vi "GetGPIBName.vi"(8 "Error In":errorcluster, 9 "GPIB ID":u32=1 min=1 step=1, 10 "GPIB Board":u32 min=1 step=1, 11 "VISA Resource List":string[](array[string])) -> (0 "Error Out":errorcluster, 2 "Found?":bool, 3 "VISA GPIB Resource Name":string)   [LabVIEW 2013, in "LV-Utilities.lvlib"]
uses:
  LV-Utilities.lvlib
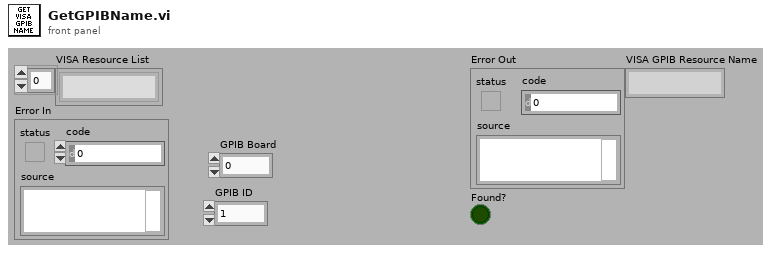
[diagram p1: front panel]
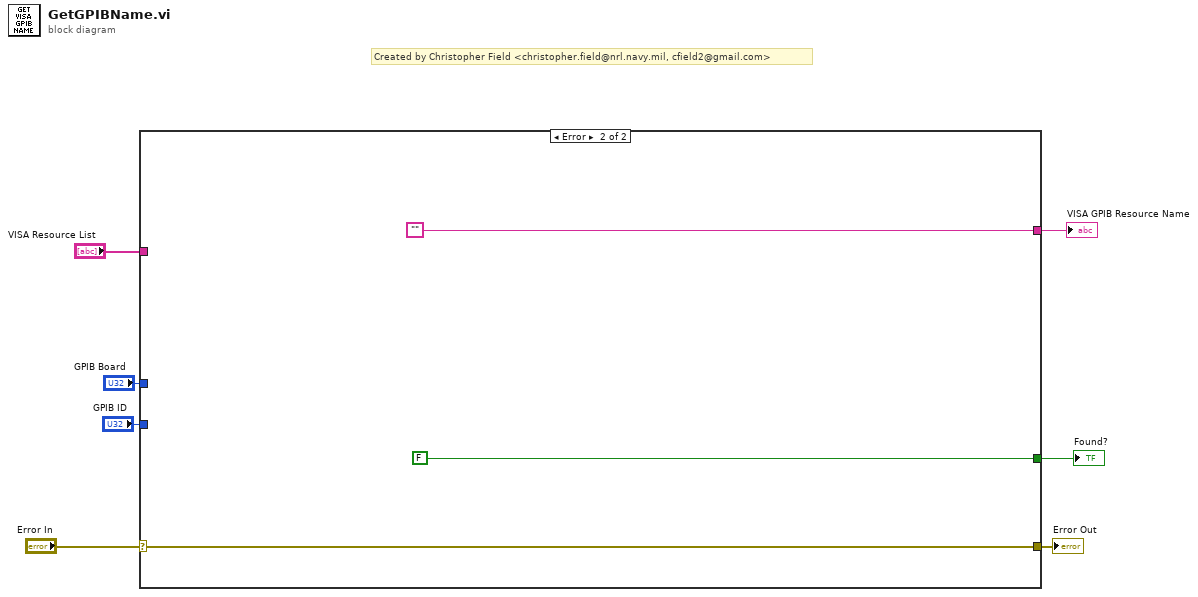
[diagram p0: block diagram]
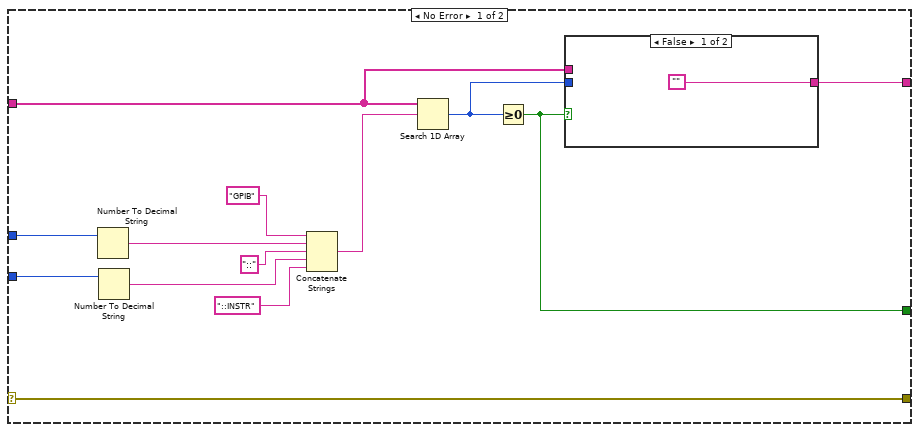
[diagram p2: hidden frame]
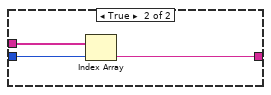
[diagram p3: hidden frame]
diagram:
  # "Created by Christopher Field <christopher.field@nrl.navy.mil, cfield2@gmail.com>"
  n1 = case shown="Error" "Error In" {
    selector: "Error In" -> [w19 w27]
    tunnel: "GPIB ID" -> [w20 _]
    tunnel: [w19 w27] -> w6
    tunnel: [w8 ""] -> w5
    tunnel: "VISA Resource List" -> [w10 _]
    tunnel: "GPIB Board" -> [w17 _]
    tunnel: [w11 FALSE] -> w1
    frame No Error {
      n2 = Number To Decimal String(number=w17) -> (decimal integer string=w16:string)  [unwired: 1 in]
      n3 = Number To Decimal String(number=w20) -> (decimal integer string=w18:string)  [unwired: 1 in]
      n4 = Concatenate Strings("GPIB" ("regular expression"), w16, "::" ("regular expression"), w18, "::INSTR" ("regular expression")) -> (w12:string)
      n5 = Search 1D Array(1D array=w10, element=w12) -> (index of element=w9:i32)  [unwired: 1 in]
      n6 = Greater Or Equal To 0?(x=w9) -> (x >= 0?=w11:bool)
      n7 = case shown="False" w11 {
        tunnel: w10 -> [_ w24]
        tunnel: w9 -> [_ w23]
        tunnel: ["" w22] -> w8
        frame False {
        }
        frame True {
          n8 = Index Array(array=w24, index=w23) -> (element=w22:string)
        }
      }
    }
    frame Error {
    }
  }
  "Error Out" <- w6
  "VISA GPIB Resource Name" <- w5
  "Found?" <- w1
